vi "check diagnostics.vi"(8 "error in":errorcluster, 10 "data dictionary in":refnum<class "data dictionary.lvclass">, 11 "Profibus Module configuration in":refnum<class "Profibus Module configuration.lvclass">) -> (0 "error out":errorcluster, 3 "diagnostics":T1[](array[typedef]))   [LabVIEW 2013, in "Profibus Module runtime.lvclass"]
uses:
  Profibus Module runtime.lvclass
  <vilib>/NI/Tag Bus/dictionary/data dictionary.lvclass
  configuration/Profibus Module configuration.lvclass
  profibus diagnostics reporting.ctl
  configuration/error throw specification.ctl
  configuration/Profibus Module configuration.lvclass/Profibus Module configuration.ctl
  <vilib>/NI/Tag Bus/tag/tag descriptor.lvclass/tag descriptor.ctl
  <vilib>/NI/Tag Bus/dictionary/data dictionary.lvclass/data dictionary.ctl
  <vilib>/NI/Tag Bus/dictionary/lookup polymorphs/locate Array of U8.vi
  <vilib>/NI/Tag Bus/dictionary/search/find data index.vi
  <vilib>/NI/Tag Bus/dictionary/search/search string list.vi
  <vilib>/NI/Tag Bus/dictionary/tag not found.vi
  <vilib>/NI/Tag Bus/tag/tag descriptor.lvclass
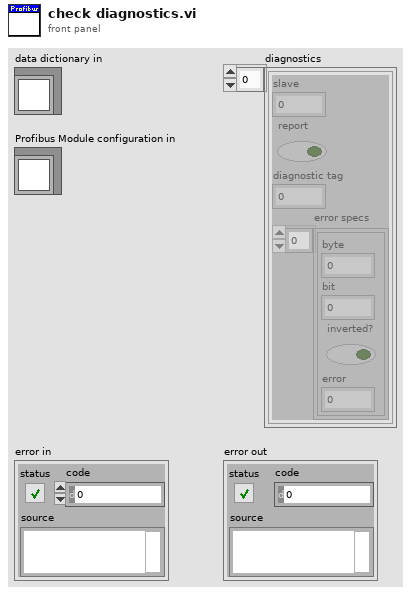
[diagram p1: front panel]
types:
  T1 = typedef "Profibus Module runtime.lvclass/profibus diagnostics reporting.ctl" = cluster{"slave":i8, "report":bool, "diagnostic tag":i32, "error specs":T2[]}
  T2 = typedef "Profibus Module configuration.lvclass/error throw specification.ctl" = cluster{"byte":i32, "bit":i32, "inverted?":bool, "error":i32}
  T3 = typedef "Profibus Module configuration.lvclass/slave diagnostic configuration.ctl" = cluster{"slave":i8, "report":bool, "channel":refnum<class "TBM channel.lvclass">, "error specs":T2[]}
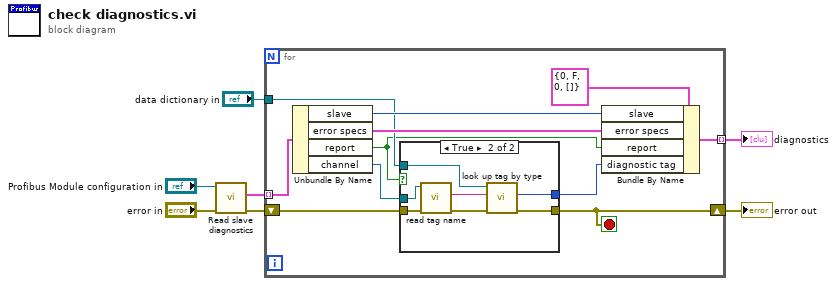
[diagram p0: block diagram]
diagram:
  n1 = call "Read slave diagnostics.vi"("error in"="error in", "Profibus Module configuration in"="Profibus Module configuration in") -> ("error out"=w4:errorcluster, "slave diagnostics"=w5:T3[])  [unwired: 7 in, 1 out]
  n2 = for {
    tunnel: w5 -> [w18] mode=indexing
    shift-right: [w9] -> w3
    shift-left: w4 -> [w13]
    tunnel: [w16] -> w2 mode=indexing
    tunnel: "data dictionary in" -> [w11]
    stop <- w9 stop-if-true
    n3 = Unbundle By Name(w18) -> ("slave"=w14:i8, "error specs"=w15:T2[], "report"=w8:bool, "channel"=w12:refnum<class "TBM channel.lvclass">)
    n4 = case shown="True" w8 {
      tunnel: w13 -> [w19 w23]
      tunnel: w12 -> [_ w22]
      tunnel: w11 -> [_ w26]
      tunnel: [w19 w25] -> w9
      tunnel: [_ w24] -> w10
      frame False {
      }
      frame True {
        n5 = call <vilib>:"read tag name.vi"("error in"=w23, "system tag in"=w22) -> ("error out"=w21:errorcluster, "name"=w20:string)  [unwired: 7 in, 1 out]
        n6 = call-poly <vilib>:"look up tag by type.vi"("error in"=w21, "name"=w20, "data dictionary in"=w26) -> ("error out"=w25:errorcluster, "index"=w24:i32)  [unwired: 6 in, 1 out]
      }
    }
    n7 = Bundle By Name(cluster=T1 {"slave"=0, "report"=FALSE, "diagnostic tag"=0, "error specs"=[]} ("diagnostics settings"), "slave"=w14, "error specs"=w15, "report"=w8, "diagnostic tag"=w10) -> (w16:T1)
  }
  "diagnostics" <- w2
  "error out" <- w3
